vi "myRIO_BRig_RT_dataLC_Cue1_Probability_NS_l1.vi"() -> (2 "output_Cue1_l1_All_Probability":i32)   [LabVIEW 2014]
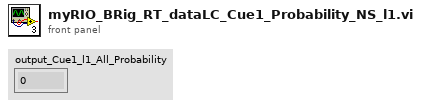
[diagram p1: front panel]
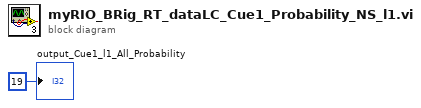
[diagram p0: block diagram]
diagram:
  "output_Cue1_l1_All_Probability" <- 19 ("output_iBlock")
